vi "Configure Continuous Sweep.vi"(0 "template configuration":refnum<class "SV Signal.lvclass">, 1 "amplitude":dbl=1.0, 5 "frequency range [Hz]":cluster{"start":dbl, "stop":dbl}={"start"=10.0, "stop"=10000.0} {"stop" format="%.2f"; "start" format="%.2f"}, 7 "duration [s]":dbl=1.0, 9 "profile":u16(ring)=1 items=["Linear", "Logarithmic"], 11 "error in (no error)":errorcluster) -> (4 "signal configuration":refnum<class "SV Continuous Sweep.lvclass">, 15 "error out":errorcluster)   [LabVIEW 2017, in "SV Continuous Sweep.lvclass"]
doc: "Configures a user-defined test signal. Wire the outputs to SV Signal (waveform) VI to generate the test signal, or wire to SV Signal Property Node to configure additional parameters before wiring to the SV Signal (waveform) VI."
uses:
  <vilib>/addons/_NISVFA/_Generation/Signal Generation/SV Continuous Sweep/SV Continuous Sweep.lvclass
  C:/Program Files (x86)/National Instruments/LabVIEW 2017/vi.lib/addons/_NISVFA/_Generation/Signal Generation/SV Signal/SV Signal.lvclass
  <vilib>/addons/_NISVFA/_Generation/Signal Generation/SV Signal/SV Signal.lvclass
  <vilib>/addons/_NISVFA/_Generation/Signal Generation/SV Signal/sv_System Timing Model.ctl
  <vilib>/addons/_NISVFA/_Generation/Signal Generation/SV Continuous Sweep/SV Continuous Sweep.lvclass/SV Continuous Sweep.ctl
  <vilib>/addons/_NISVFA/_Generation/Signal Generation/SV Signal/Write System Timing Model.vi
  <vilib>/addons/_NISVFA/_Generation/Signal Generation/SV Signal/Write Measurement Duration.vi
  <vilib>/addons/_NISVFA/_Generation/Signal Generation/SV Signal/Write Sample Rate.vi
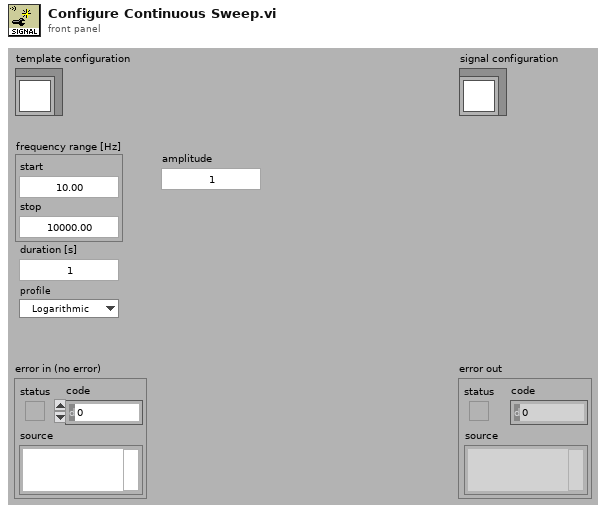
[diagram p1: front panel]
types:
  T1 = typedef "SV Signal.lvclass/sv_System Timing Model.ctl" = i64
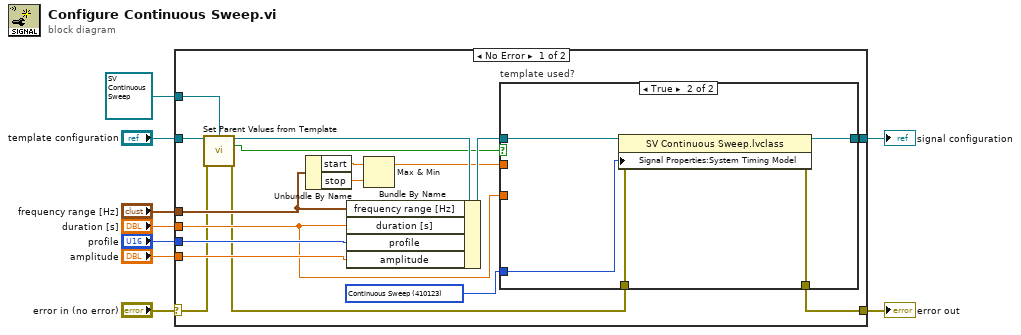
[diagram p0: block diagram]
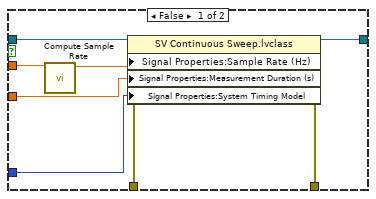
[diagram p2: hidden frame]
diagram:
  n1 = case shown="No Error" "error in (no error)" {
    selector: "error in (no error)" -> [w15 w40]
    tunnel: [w13 w40] -> w8
    tunnel: [w23 w41] -> w6
    tunnel: refnum<class "SV Continuous Sweep.lvclass"> refnum ("ContinuousSweep in") -> [w17 w41]
    tunnel: "frequency range [Hz]" -> [w21 _]
    tunnel: "duration [s]" -> [w22 _]
    tunnel: "profile" -> [w26 _]
    tunnel: "amplitude" -> [w25 _]
    tunnel: "template configuration" -> [w18 _]
    frame No Error {
      w10 = T1 410123 items=["Finite"=10178, "-"=-1, "Continuous"=10123, "-"=-2, "Settled"=110123, "Averaged"=210123, "Discrete Sweep"=310123, "Continuous Sweep"=410123] ("System Timing Model")
      n2 = call-dynamic "Set Parent Values from Template.vi"("template configuration"=w18, "signal configuration in"=w17, "error in (no error)"=w15) -> ("signal configuration out"=w16:refnum<class "SV Continuous Sweep.lvclass">, "template used?"=w11:bool, "error out"=w14:errorcluster)  [unwired: 10 in]
      n3 = Unbundle By Name(w21) -> ("start"=w20:dbl, "stop"=w19:dbl)
      n4 = Bundle By Name(cluster=w16, "frequency range [Hz]"=w21, "duration [s]"=w22, "profile"=w26, "amplitude"=w25) -> (w24:refnum<class "SV Continuous Sweep.lvclass">)
      n5 = Max & Min(x=w20, y=w19) -> (max(x,y)=w12:dbl)  [unwired: 1 out]
      n6 = case "template used?" shown="True" w11 {
        tunnel: w24 -> [w34 w39]
        tunnel: [w33 w38] -> w23
        tunnel: w22 -> [w32 _]
        tunnel: w12 -> [w29 _]
        tunnel: w14 -> [w31 w37]
        tunnel: [w30 w36] -> w13
        tunnel: w10 -> [w27 w35]
        frame False {
          n7 = call <vilib>:"Compute Sample Rate.vi"("maximum frequency [Hz]"=w29) -> ("sample rate [Hz]"=w28:dbl)  [unwired: 10 in]
          n8 = property class="SV Continuous Sweep.lvclass"(reference=w34, error in=w31, "Signal Properties:Sample Rate (Hz)"=w28, "Signal Properties:Measurement Duration (s)"=w32, "Signal Properties:System Timing Model"=w27) -> (reference out=w33:refnum<class "SV Continuous Sweep.lvclass">, error out=w30:errorcluster)
        }
        frame True {
          n9 = property class="SV Continuous Sweep.lvclass"(reference=w39, error in=w37, "Signal Properties:System Timing Model"=w35) -> (reference out=w38:refnum<class "SV Continuous Sweep.lvclass">, error out=w36:errorcluster)
        }
      }
    }
    frame Error {
    }
  }
  "error out" <- w8
  "signal configuration" <- w6
